vi "Set Value.vi"(8 "error in (no error)":errorcluster, 10 "Project Info Value":string, 11 "Timestamp Item Configuration in":refnum<class "Timestamp Item Configuration.lvclass">) -> (0 "error out":errorcluster, 3 "Timestamp Item Configuration out":refnum<class "Timestamp Item Configuration.lvclass">)   [LabVIEW 2013, in "Item Configuration.lvlib" / "Timestamp Item Configuration.lvclass"]
uses:
  Timestamp Item Configuration.lvclass
  <vilib>/Utility/miscctls.llb/LVDateTimeRec.ctl
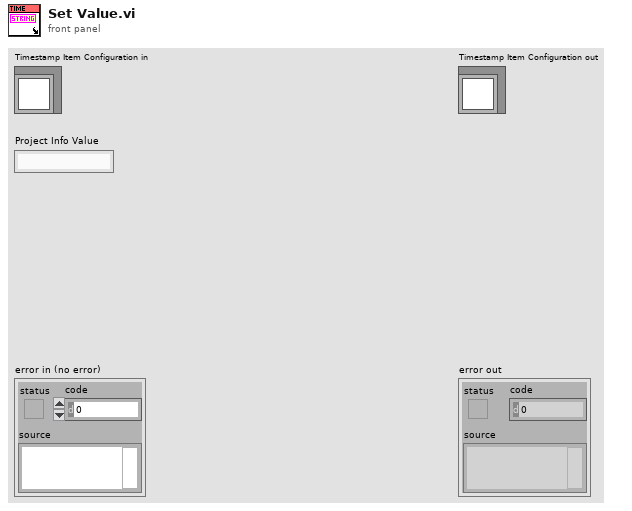
[diagram p1: front panel]
types:
  T1 = typedef "LVDateTimeRec.ctl" = cluster{"fractional second":dbl, "second":i32, "minute":i32, "hour":i32, "day of month":i32, "month":i32, "year":i32, "day of week":i32, "day of year":i32, "DST":i32}
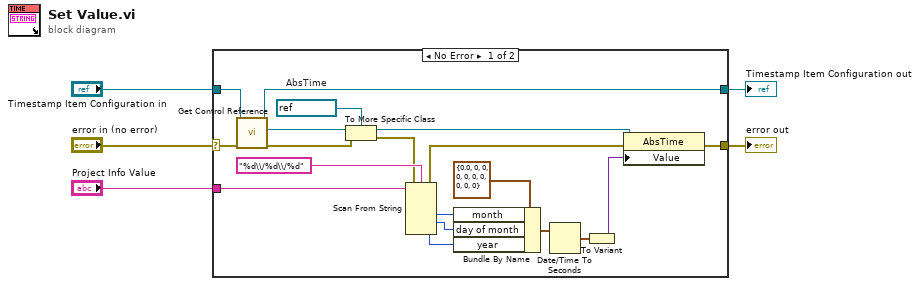
[diagram p0: block diagram]
diagram:
  n1 = case shown="No Error" "error in (no error)" {
    selector: "error in (no error)" -> [w23 w26]
    tunnel: "Timestamp Item Configuration in" -> [w24 w25]
    tunnel: "Project Info Value" -> [w16 _]
    tunnel: [w7 w26] -> w2
    tunnel: [w6 w25] -> w1
    frame No Error {
      w21 = refnum<vi> refnum  # AbsTime
      n2 = call-dynamic "Get Control Reference.vi"("error in (no error)"=w23, "Item Configuration in"=w24) -> ("error out"=w20:errorcluster, "Control Reference"=w22:refnum<vi>, "Item Configuration out"=w6:refnum<class "Timestamp Item Configuration.lvclass">)  [unwired: 7 in]
      n3 = To More Specific Class(target class=w21, reference=w22, error in=w20) -> (specific class reference=w19:refnum<vi>, error out=w10:errorcluster)
      n4 = Scan From String(format string="%d\\/%d\\/%d", input string=w16, error in=w10) -> (error out=w11:errorcluster, output 1=w13:i32, output 2=w14:i32, output 3=w15:i32)  [unwired: 4 in, 2 out]
      n5 = Bundle By Name(cluster=T1 {"fractional second"=0.0, "second"=0, "minute"=0, "hour"=0, "day of month"=0, "month"=0, "year"=0, "day of week"=0, "day of year"=0, "DST"=0} ("date time rec"), "month"=w13, "day of month"=w14, "year"=w15) -> (w12:T1)
      n6 = Date/Time To Seconds(2:w12) -> (0:w9:timestamp)  [unwired: 1 in]
      n7 = To Variant(anything=w9) -> (Variant=w8:variant)
      n8 = property class="AbsTime"(reference=w19, error in=w11, "Value"=w8) -> (error out=w7:errorcluster)  [unwired: 1 out]
    }
    frame Error {
    }
  }
  "error out" <- w2
  "Timestamp Item Configuration out" <- w1
